vi "Production inquiry.vi"() -> ()   [LabVIEW 2014]
uses:
  <vilib>/Utility/NIReport.llb/NI_report.lvclass
  <vilib>/Utility/NIReport.llb/Append Text Table to Report (wrap).vi
panel:
  out "错误输出":errorcluster
  in  "菜单下拉列表":u16(ring) items=["PA10", "PA20", "PA30", "PA50", "ST30", "ST90"]
  out "正常":bool
  out "异常":bool
  out "查询表格":string[][](table) caption="PA50"
  in  "截止时间":timestamp format="%<%H:%M:%S\n%y/%m/%d>T"
  in  "起始时间":timestamp format="%<%H:%M:%S\n%y/%m/%d>T"
  in  "退出":bool
  in  "确认扫码":bool
  in  "扫码":string
  in  "确认时间":bool
  # "已生产产品查询系统"
  # "时间格式查询："
  # "截止时间"
  # "起始时间"
  # "扫码格式查询："
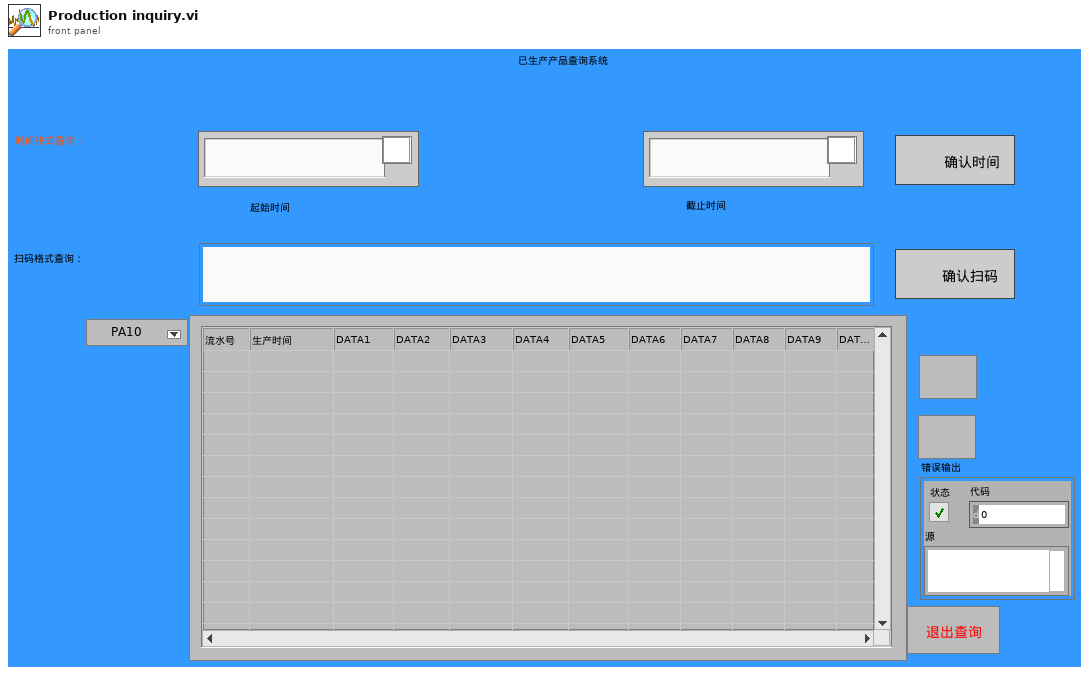
[diagram p1: front panel]
types:
  T1 = enum16{"open", "replace", "create", "open or create", "replace or create", "replace or create with confirmation"}
  T2 = enum16{"Standard Report", "HTML", "Word", "Excel"}
  T3 = cluster{"position (excel)":cluster{"row":i32, "column":i32}, "name (excel)":string, "bookmark (word)":string}
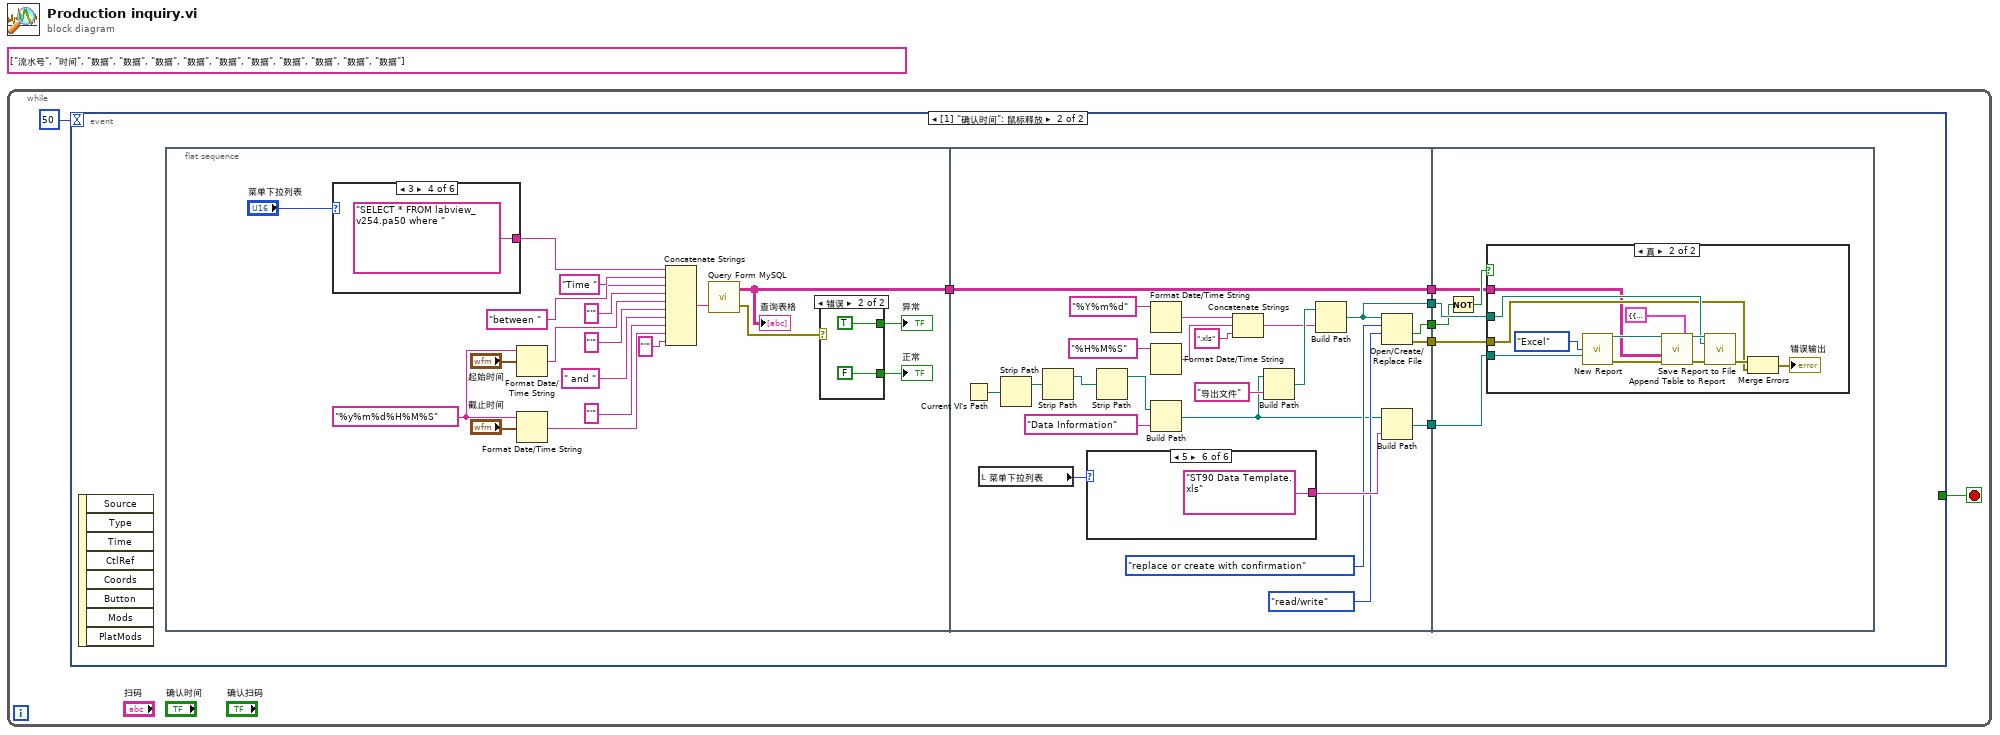
[diagram p0: block diagram]
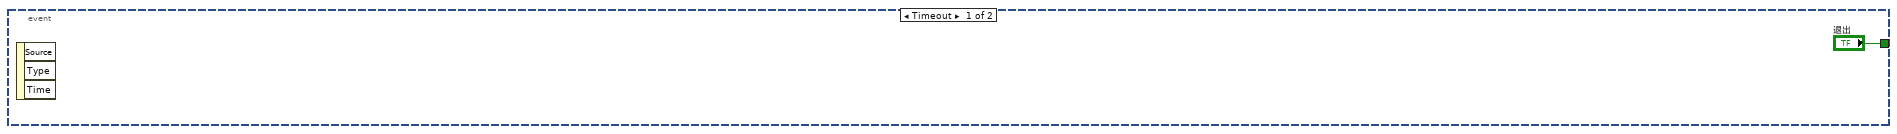
[diagram p2: hidden frame]
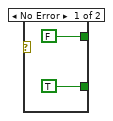
[diagram p3: hidden frame]
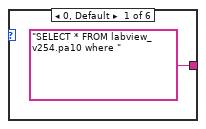
[diagram p4: hidden frame]
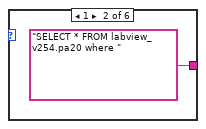
[diagram p5: hidden frame]
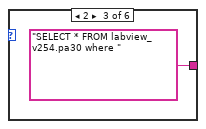
[diagram p6: hidden frame]
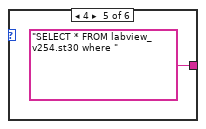
[diagram p7: hidden frame]
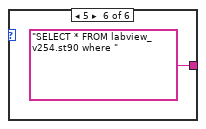
[diagram p8: hidden frame]
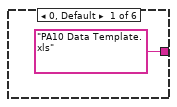
[diagram p9: hidden frame]
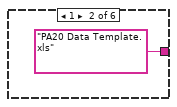
[diagram p10: hidden frame]
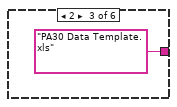
[diagram p11: hidden frame]
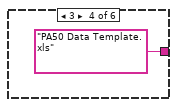
[diagram p12: hidden frame]
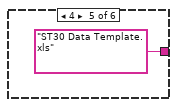
[diagram p13: hidden frame]
diagram:
  (unwired) string[] ["流水号", "时间", "数据", "数据", "数据", "数据", "数据", "数据", "数据", "数据", "数据", "数据"] ("row headers")
  n1 = while {
    stop <- w1 stop-if-true
    n2 = event shown="[1] \"确认时间\": 鼠标释放" {
      selector: _ -> [_ _]
      dyn-events: _ -> [_ _]
      timeout: 50 -> [_ _]
      tunnel: ["退出" _] -> w1
      event Timeout {
        n3 = event-data() -> ()  [unwired: 1 in, 3 out]
      }
      event "确认时间": Mouse Up {
        n4 = event-data() -> ()  [unwired: 1 in, 8 out]
        n5 = flat-sequence {
          tunnel: [w10] -> w4
          tunnel: [w55] -> w9
          tunnel: [w47] -> w8
          tunnel: [w41] -> w7
          tunnel: [w40] -> w6
          tunnel: [w39] -> w5
          tunnel: w4 -> [w39]
          tunnel: w9 -> [w73]
          tunnel: w8 -> [w72]
          tunnel: w7 -> [w71]
          tunnel: w6 -> [w70]
          tunnel: w5 -> [w68]
          frame #0 {
            w18 = "%y%m%d%H%M%S" ("时间格式字符串(%c)")
            n6 = case shown="3" "菜单下拉列表" {
              tunnel: ["SELECT * FROM labview_v254.pa10 where " ("SQL query") "SELECT * FROM labview_v254.pa20 where " ("SQL query") "SELECT * FROM labview_v254.pa30 where " ("SQL query") "SELECT * FROM labview_v254.pa50 where " ("SQL query") "SELECT * FROM labview_v254.st30 where " ("SQL query") "SELECT * FROM labview_v254.st90 where " ("SQL query")] -> w25
              frame 0, Default {
              }
              frame 1 {
              }
              frame 2 {
              }
              frame 3 {
              }
              frame 4 {
              }
              frame 5 {
              }
            }
            n7 = Format Date/Time String(time format string (%c)=w18, seconds (now)="起始时间") -> (date/time string=w27:string)  [unwired: 1 in]
            n8 = Format Date/Time String(time format string (%c)=w18, seconds (now)="截止时间") -> (date/time string=w28:string)  [unwired: 1 in]
            n9 = Concatenate Strings(w25, "Time " ("字符串"), "between " ("输入 2"), "'" ("字符串"), w27, "'" ("字符串"), " and " ("字符串"), "'" ("字符串"), w28, "'" ("字符串")) -> (w26:string)
            n10 = call "Query Form MySQL.vi"("SQL query"=w26) -> ("error out"=w23:errorcluster, "data"=w10:string[][])  [unwired: 1 in]
            "查询表格" <- w10
            n11 = case shown="错误" w23 {
              tunnel: [FALSE ("异常") TRUE ("异常")] -> w22
              tunnel: [TRUE ("正常") FALSE ("正常")] -> w21
              frame No Error {
              }
              frame Error {
              }
            }
            "正常" <- w21
            "异常" <- w22
          }
          frame #1 {
            n12 = Current VI's Path() -> (path=w59:path)
            n13 = local read "菜单下拉列表"() -> (w57:u16)
            n14 = Strip Path(path=w59) -> (stripped path=w60:path)  [unwired: 1 out]
            n15 = Strip Path(path=w60) -> (stripped path=w61:path)  [unwired: 1 out]
            n16 = case shown="5" w57 {
              tunnel: ["PA10 Data Template.xls" ("名称或相对路径") "PA20 Data Template.xls" ("名称或相对路径") "PA30 Data Template.xls" ("名称或相对路径") "PA50 Data Template.xls" ("名称或相对路径") "ST30 Data Template.xls" ("名称或相对路径") "ST90 Data Template.xls" ("名称或相对路径")] -> w56
              frame 0, Default {
              }
              frame 1 {
              }
              frame 2 {
              }
              frame 3 {
              }
              frame 4 {
              }
              frame 5 {
              }
            }
            n17 = Strip Path(path=w61) -> (stripped path=w54:path)  [unwired: 1 out]
            n18 = Format Date/Time String(time format string (%c)="%Y%m%d" ("时间格式字符串(%c)")) -> (date/time string=w43:string)  [unwired: 2 in]
            n19 = Format Date/Time String(time format string (%c)="%H%M%S" ("时间格式字符串(%c)")) -> (date/time string=w42:string)  [unwired: 2 in]
            n20 = Build Path(base path=w54, name or relative path="Data Information" ("名称或相对路径")) -> (appended path=w46:path)
            n21 = Concatenate Strings(w43, w42, ".xls" ("字符串")) -> (w50:string)
            n22 = Build Path(base path=w46, name or relative path="导出文件" ("名称或相对路径")) -> (appended path=w52:path)
            n23 = Build Path(base path=w52, name or relative path=w50) -> (appended path=w47:path)
            n24 = Open/Create/Replace File(file path (use dialog)=w47, operation (0:open)=T1."replace or create with confirmation" ("操作(0:open)"), access (0:read/write)=enum16{"read/write", "read-only", "write-only"}."read/write" ("权限(0:read/write)")) -> (cancelled=w40:bool, error out=w41:errorcluster)  [unwired: 3 in, 1 out]
            n25 = Build Path(base path=w46, name or relative path=w56) -> (appended path=w55:path)
          }
          frame #2 {
            n26 = Not(x=w70) -> (.not. x?=w69:bool)
            n27 = case shown="真" w69 {
              tunnel: w73 -> [_ w77]
              tunnel: w72 -> [_ w76]
              tunnel: w71 -> [_ w75]
              tunnel: w68 -> [_ w74]
              frame False {
              }
              frame True {
                n28 = call <vilib>:"New Report.vi"("report type"=T2."Excel", "template (empty)"=w77) -> ("report out"=w78:refnum<class "NI_report.lvclass">, "error out"=w80:errorcluster)  [unwired: 12 in]
                n29 = call-poly <vilib>:"Append Table to Report.vi"("report in"=w78, "MS Office parameters"=T3 {"position (excel)"={"row"=2, "column"=0}, "name (excel)"="", "bookmark (word)"=""}, "text data"=w74, "error in (no error)"=w80) -> ("report out"=w82:refnum<class "NI_report.lvclass">, "error out"=w83:errorcluster)  [unwired: 8 in, 2 out]
                n30 = call-dynamic "Save Report to File.vi"("report in"=w82, "report file path"=w76, "error in (no error)"=w83) -> ("error out"=w84:errorcluster)  [unwired: 11 in, 1 out]
                n31 = Merge Errors(w84, w75) -> (→"错误输出":errorcluster)
              }
            }
          }
        }
      }
    }
  }
